vi "CCD Waiting for SRQ.vi"(4 "Exposuretime (s)":dbl=0.5 format="%.2f", 5 "error in":errorcluster, 6 "time loop constant":u32, 7 "poll status waiting for":i16, 8 "GPIB Address":i16=1 min=1 max=1) -> (0 "error out":errorcluster, 1 "Poll Status":bool[](array[boolean]), 2 "Error":bool, 3 "Poll Byte":i16=65)   [LabVIEW 2024]
uses:
  Globals and TypeDefs/Error Categories.ctt
  <vilib>/Utility/error.llb/DialogType.ctl
  Globals and TypeDefs/Type Definitions.llb/3 way Status.ctl
  Globals and TypeDefs/gDetector.vi
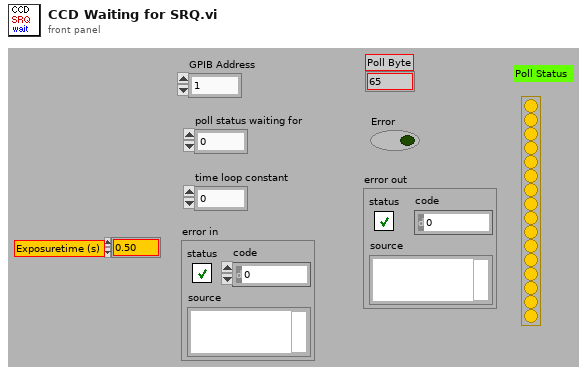
[diagram p1: front panel]
types:
  T1 = enum16{"Poll CCD GPIB Status", "Check CCD Command Error", "CheckSRQ-Poll"}
  T2 = enum8{"Initialization Error", "Command Error", "Parameter Error", "Overflow Error", "Time-out Error", "Misc Error", "User cancel"}
  T3 = typedef "Error Categories.ctt" = enum8{"General", "CCD-256x1024", "CCD-1340x400", "InGaAs PDA", "McPherson 2075", "Magnetic Field", "Temperature Control", "Other"}
  T4 = typedef "3 way Status.ctl" = u8
  T5 = typedef "DialogType.ctl" = u16
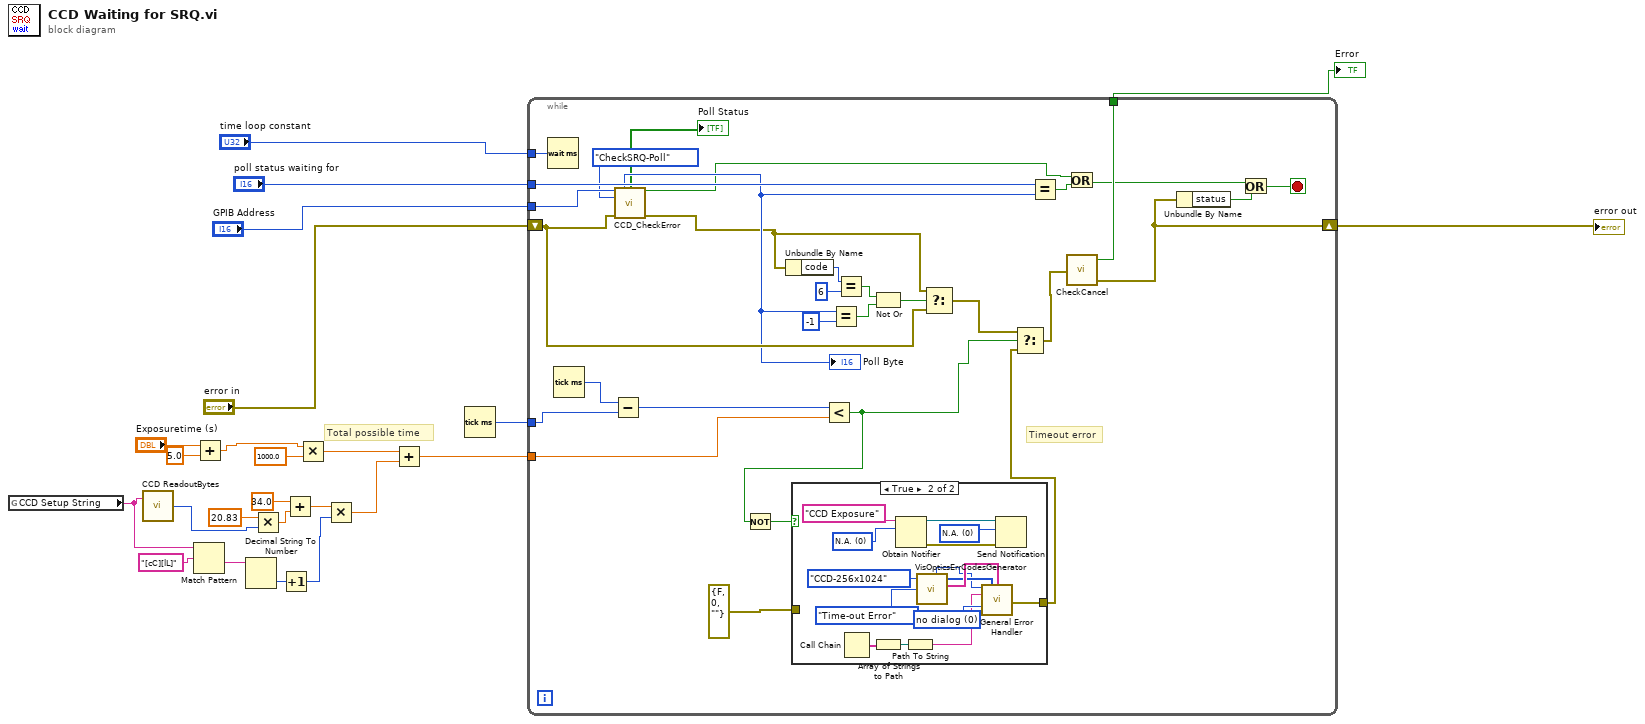
[diagram p0: block diagram]
diagram:
  # "Total possible time"
  n1 = global read "gDetector.vi" "CCD Setup String"() -> (w4:string)
  n2 = call "CCD ReadoutBytes.vi"("CCD Setup String"=w4) -> ("LD Bytes"=w13:i32)  [unwired: 1 in, 3 out]
  n3 = Match Pattern(string=w4, regular expression="[cC][lL]") -> (after substring=w3:string)  [unwired: 1 in, 3 out]
  n4 = Add(x="Exposuretime (s)", y=5.0) -> (x+y=w8:dbl)
  n5 = Decimal String To Number(string=w3) -> (number=w2:i32)  [unwired: 2 in, 1 out]
  n6 = Multiply(x=20.83, y=w13) -> (x*y=w17:dbl)
  n7 = Increment(x=w2) -> (x+1=w1:i32)
  n8 = Add(x=34.0, y=w17) -> (x+y=w12:dbl)
  n9 = Multiply(x=w8, y=1000.0) -> (x*y=w14:dbl)
  n10 = Multiply(x=w12, y=w1) -> (x*y=w11:dbl)
  n11 = Add(x=w14, y=w11) -> (x+y=w9:dbl)
  n12 = Tick Count (ms)() -> (millisecond timer value=w10:u32)
  n13 = while {
    tunnel: "GPIB Address" -> [w36]
    shift-right: [w52] -> w19
    shift-left: "error in" -> [w37]
    tunnel: "poll status waiting for" -> [w53]
    tunnel: [w51] -> w23
    tunnel: "time loop constant" -> [w50]
    tunnel: w10 -> [w43]
    tunnel: w9 -> [w40]
    stop <- w55 stop-if-true
    # "Timeout error"
    n14 = Wait (ms)(milliseconds to wait=w50) -> ()  [unwired: 1 out]
    n15 = Tick Count (ms)() -> (millisecond timer value=w44:u32)
    n16 = Subtract(x=w44, y=w43) -> (x-y=w41:u32)
    n17 = call "CCD_CheckError.vi"("CCD GPIB Address"=w36, "Mode"=T1."CheckSRQ-Poll", "error in"=w37) -> ("Poll Byte"=w34:i16, "Poll Status"=→"Poll Status":bool[], "SRQ"=w30:bool, "error out"=w33:errorcluster)  [unwired: 4 in, 5 out]
    "Poll Byte" <- w34
    n18 = Unbundle By Name(w33) -> ("code"=w48:i32)
    n19 = Less?(x=w41, y=w40) -> (x < y?=w25:bool)
    n20 = Not(x=w25) -> (.not. x?=w26:bool)
    n21 = case shown="True" w26 {
      tunnel: [w56 w66] -> w28
      tunnel: errorcluster {"status"=FALSE, "code"=0, "source"=""} ("error out") -> [w56 _]
      frame False {
      }
      frame True {
        w57 = T4 0 items=["N.A.", "OK", "Busy", "Done"] ("notification")
        w61 = T4 0 items=["N.A.", "OK", "Busy", "Done"] ("Saving")
        w71 = T5 0 items=["no dialog", "OK message", "continue or stop message", "OK message + warnings", "continue/stop + warnings"] ("type of dialog (OK msg:1)")
        n22 = Call Chain() -> (call chain=w64:string[])
        n23 = Array of Strings to Path(0:w64) -> (2:w63:path)  [unwired: 1 in]
        n24 = Obtain Notifier(name (unnamed)="CCD Exposure", notification data type=w61) -> (notifier out=w59:refnum<notifier>, error out=w58:errorcluster)  [unwired: 2 in, 1 out]
        n25 = Path To String(path=w63) -> (string=w62:string)
        n26 = call "VisOpticsErrCodesGenerator.vi"("NHMFL Visible Optics Error Type"=T2."Time-out Error", "NHMFL Visible Optics Error Categories"=Error_Categories.ctt."CCD-256x1024") -> ("user-defined descriptions"=w70:string[], "User-defined Error Code"=w65:i32, "user-defined codes"=w69:i32[])  [unwired: 1 in, 3 out]
        n27 = call <vilib>:"General Error Handler.vi"("[error code] (0)"=w65, "[user-defined codes]"=w69, "[user-defined descriptions]"=w70, "[error source] (\" \")"=w62, "type of dialog (OK msg:1)"=w71) -> ("error out"=w66:errorcluster)  [unwired: 6 in, 4 out]
        n28 = Send Notification(notification=w57, notifier=w59, error in (no error)=w58) -> ()  [unwired: 2 out]
      }
    }
    n29 = Equal?(x=w34, y=i16 -1) -> (x = y?=w45:bool)
    n30 = Equal?(x=w48, y=6) -> (x = y?=w46:bool)
    n31 = Not Or(1:w45, 2:w46) -> (0:w42:bool)
    n32 = Select(t=w33, s=w42, f=w37) -> (s? t:f=w39:errorcluster)
    n33 = Select(t=w39, s=w25, f=w28) -> (s? t:f=w38:errorcluster)
    n34 = Equal?(x=w53, y=w34) -> (x = y?=w32:bool)
    n35 = Or(x=w30, y=w32) -> (x .or. y?=w31:bool)
    n36 = call "CheckCancel.vi"("error in (no error)"=w38) -> ("Cancelled"=w51:bool, "error out"=w52:errorcluster)  [unwired: 1 in]
    n37 = Unbundle By Name(w52) -> ("status"=w54:bool)
    n38 = Or(x=w31, y=w54) -> (x .or. y?=w55:bool)
  }
  "error out" <- w19
  "Error" <- w23
